vi "Status Bar Test.vi"   [LabVIEW 2015]
uses:
  Globals.vi
  Actors/Status Bar/API/Status Bar Actor API.lvclass
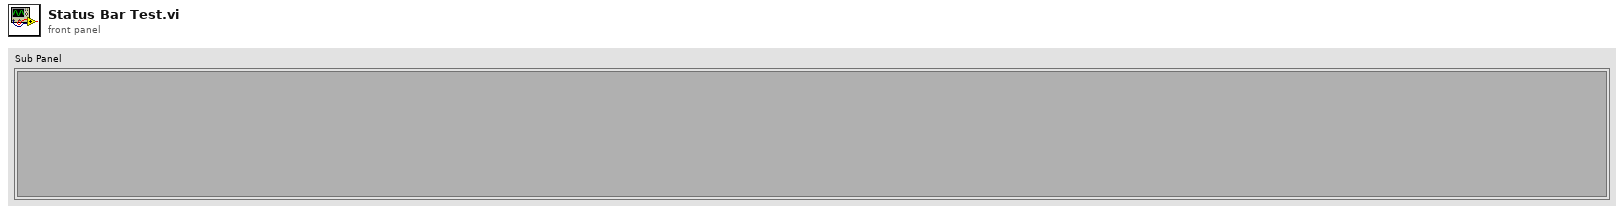
[diagram p1: front panel]
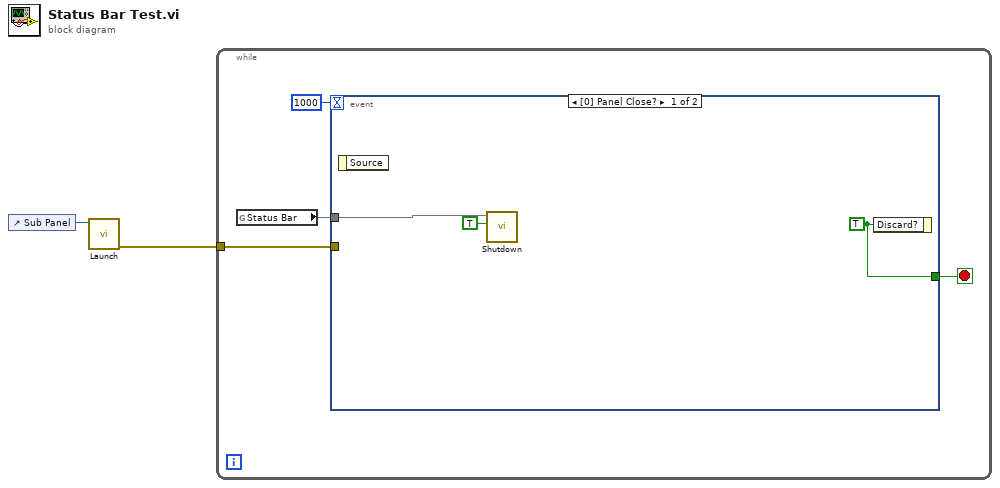
[diagram p0: block diagram]
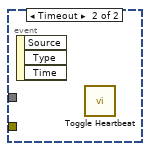
[diagram p2: hidden frame]
diagram:
  n1 = control-ref of="Sub Panel"() -> (w2:refnum<vi>)
  n2 = call "Launch.vi"("Sub Panel"=w2) -> ("error out"=w1:errorcluster)  [unwired: 9 in, 1 out]
  n3 = while {
    tunnel: w1 -> [w4]
    stop <- w6 stop-if-true
    n4 = global read "Globals.vi" "Status Bar"() -> (w3)
    n5 = event shown="[0] Panel Close?" {
      selector: _ -> [_ _]
      dyn-events: _ -> [_ _]
      timeout: 1000 -> [_ _]
      tunnel: [w9 _] -> w6
      tunnel: w4 -> [_ _]
      tunnel: w3 -> [w7 _]
      event Panel Close? {
        w9 = TRUE ("Discard?")
        n6 = event-data() -> ()  [unwired: 1 in, 1 out]
        n7 = call-dynamic "Shutdown.vi"("Wait For Shutdown (F)"=TRUE, "Actor API in"=w7) -> ()  [unwired: 9 in, 1 out]
        n8 = event-data("Discard?"=w9) -> ()  [unwired: 1 in, 1 out]
      }
      event Timeout {
        n9 = event-data() -> ()  [unwired: 1 in, 3 out]
        n10 = call "Toggle Heartbeat.vi"() -> ()  [unwired: 11 in, 1 out]
      }
    }
  }
